vi "Execute.vi"(8 "error in (no error)":errorcluster, 10 "Plugin Handler Launch Plugin in":refnum<class "Plugin Handler Launch Plugin.lvclass">, 11 "Plugin Handler Shifter Data Definition":T1) -> (0 "error out":errorcluster, 1 "Stop?":bool, 2 "Plugin Generic Command out":refnum<class "Plugin Handler Command.lvclass">, 3 "Plugin Handler Shifter Data Out":T1)   [LabVIEW 2011, in "Plugin Handler Launch Plugin.lvclass"]
uses:
  Plugin Handler Launch Plugin.lvclass
  Plugin Handler Command.lvclass
  Plugin Strict Type Definitions/Plugin Handler Shifter Data Definition.ctl
  Parent Plugin Definition/Plugin Template/Generic Plugin.lvclass
  Plugin Strict Type Definitions/Plugin Configuration Information.ctl
  User Interface/UI Command Manager/UI Command Manager.lvclass
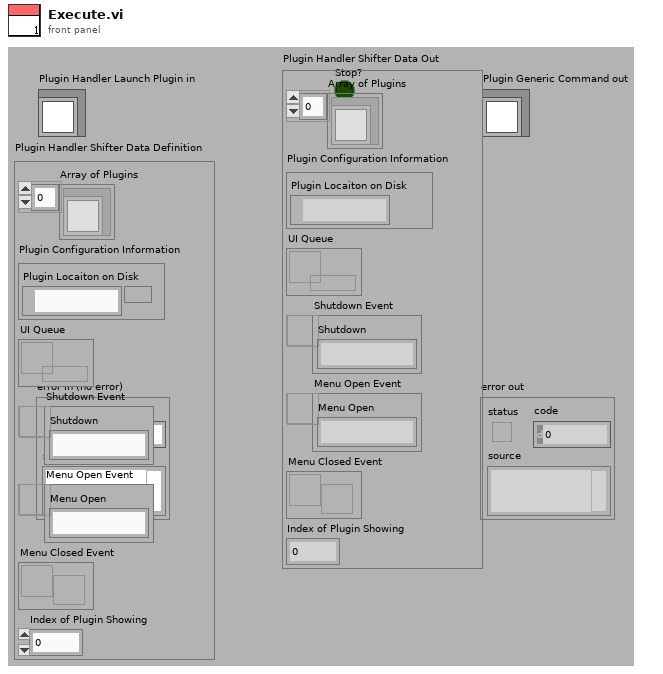
[diagram p1: front panel]
types:
  T1 = typedef "Plugin Handler Shifter Data Definition.ctl" = cluster{"Array of Plugins":refnum<class "Generic Plugin.lvclass">[], "Plugin Configuration Information":T2, "UI Queue":refnum<queue>, "Shutdown Event":refnum<user-event>, "Menu Open Event":refnum<user-event>, "Menu Closed Event":refnum<user-event>, "Index of Plugin Showing":i32}
  T2 = typedef "Plugin Configuration Information.ctl" = cluster{"Plugin Locaiton on Disk":path}
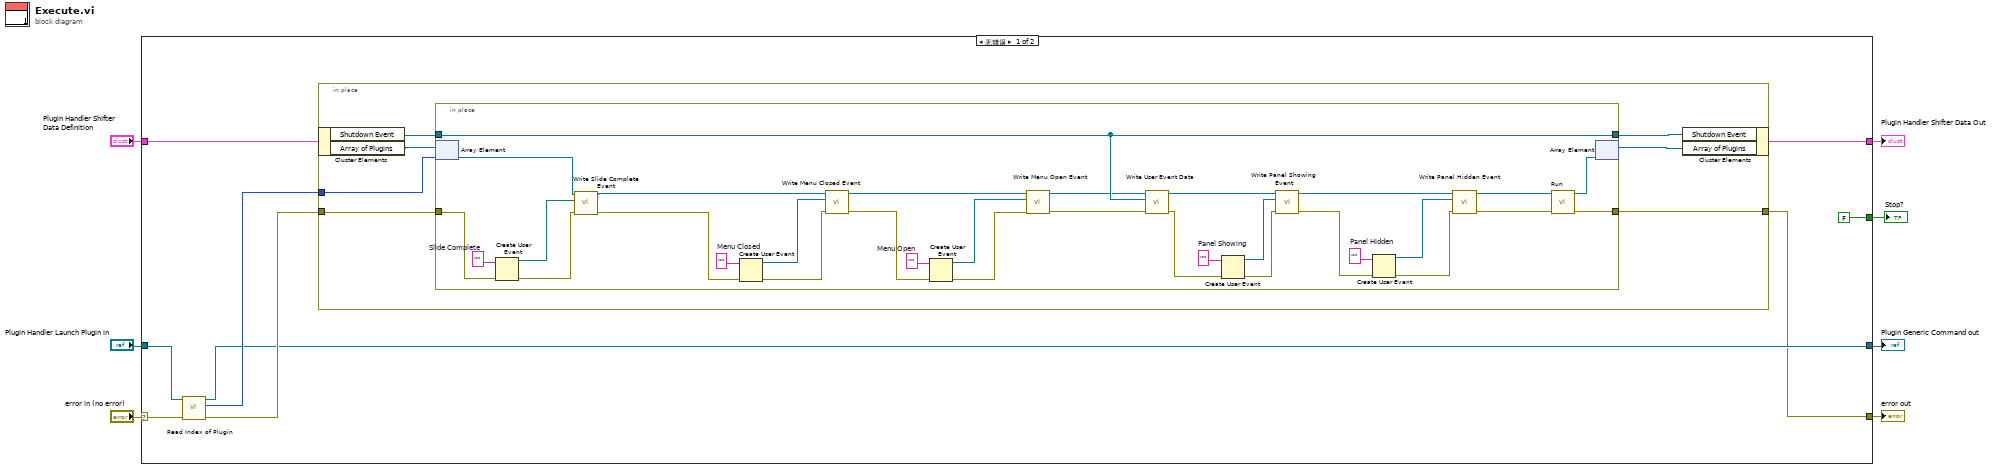
[diagram p0: block diagram]
diagram:
  n1 = case shown="无错误" "error in (no error)" {
    selector: "error in (no error)" -> [w13 w58]
    tunnel: "Plugin Handler Launch Plugin in" -> [w16 w57]
    tunnel: "Plugin Handler Shifter Data Definition" -> [w10 w56]
    tunnel: [w9 w56] -> w5
    tunnel: [w11 w58] -> w3
    tunnel: [w12 w57] -> w2
    tunnel: [FALSE ("Stop?") _] -> w1
    frame No Error {
      n2 = call-dynamic "Read Index of Plugin.vi"("error in (no error)"=w13, "Plugin Handler Launch Plugin in"=w16) -> ("error out"=w14:errorcluster, "Index of Plugin"=w15:i32, "Plugin Handler Launch Plugin out"=w12:refnum<class "Plugin Handler Launch Plugin.lvclass">)  [unwired: 7 in]
      n3 = in-place {
        in-place-border: w15 -> [w20]
        in-place-border: w14 -> [w23]
        in-place-border: [w22] -> w11
        n4 = in-place-cluster #1(w10) -> ("Shutdown Event"=w21:refnum<user-event>, "Array of Plugins"=w18:refnum<class "Generic Plugin.lvclass">[])
        n5 = in-place {
          in-place-border: w23 -> [w32]
          in-place-border: [w50] -> w22
          in-place-border: w21 -> [w55]
          in-place-border: [w55] -> w19
          w33 = ""  # Slide Complete
          w37 = ""  # Menu Open
          w40 = ""  # Menu Closed
          w48 = ""  # Panel Hidden
          w54 = ""  # Panel Showing
          n6 = in-place-array #2(w18, w20) -> (w30:refnum<class "Generic Plugin.lvclass">)
          n7 = Create User Event(user event datatype=w33, error in=w32) -> (user event=w31:refnum<user-event>, error out=w28:errorcluster)
          n8 = call "Write Slide Complete Event.vi"("error in (no error)"=w28, "Slide Complete Event"=w31, "Generic Plugin in"=w30) -> ("error out"=w27:errorcluster, "Generic Plugin out"=w29:refnum<class "Generic Plugin.lvclass">)  [unwired: 7 in]
          n9 = Create User Event(user event datatype=w40, error in=w27) -> (user event=w39:refnum<user-event>, error out=w38:errorcluster)
          n10 = call "Write Menu Closed Event.vi"("error in (no error)"=w38, "Menu Closed Event"=w39, "Generic Plugin in"=w29) -> ("error out"=w35:errorcluster, "Generic Plugin out"=w41:refnum<class "Generic Plugin.lvclass">)  [unwired: 7 in]
          n11 = Create User Event(user event datatype=w37, error in=w35) -> (user event=w36:refnum<user-event>, error out=w34:errorcluster)
          n12 = call "Write Menu Open Event.vi"("error in (no error)"=w34, "Menu Open Event"=w36, "Generic Plugin in"=w41) -> ("error out"=w25:errorcluster, "Generic Plugin out"=w42:refnum<class "Generic Plugin.lvclass">)  [unwired: 7 in]
          n13 = call "Write User Event Data.vi"("error in (no error)"=w25, "User Event Data"=w55, "Generic Plugin in"=w42) -> ("error out"=w24:errorcluster, "Generic Plugin out"=w52:refnum<class "Generic Plugin.lvclass">)  [unwired: 7 in]
          n14 = Create User Event(user event datatype=w54, error in=w24) -> (user event=w53:refnum<user-event>, error out=w26:errorcluster)
          n15 = call "Write Panel Showing Event.vi"("error in (no error)"=w26, "Panel Showing Event"=w53, "Generic Plugin in"=w52) -> ("error out"=w47:errorcluster, "Generic Plugin out"=w49:refnum<class "Generic Plugin.lvclass">)  [unwired: 7 in]
          n16 = Create User Event(user event datatype=w48, error in=w47) -> (user event=w45:refnum<user-event>, error out=w44:errorcluster)
          n17 = call "Write Panel Hidden Event.vi"("error in (no error)"=w44, "Panel Hidden Event"=w45, "Generic Plugin in"=w49) -> ("error out"=w43:errorcluster, "Generic Plugin out"=w46:refnum<class "Generic Plugin.lvclass">)  [unwired: 7 in]
          n18 = call-dynamic "Run.vi"("error in (no error)"=w43, "Generic Plugin in"=w46) -> ("error out"=w50:errorcluster, "Generic Plugin out"=w51:refnum<class "Generic Plugin.lvclass">)  [unwired: 8 in]
          n19 = in-place-array #2(w51) -> (w17:refnum<class "Generic Plugin.lvclass">[])  [unwired: 1 out]
        }
        n20 = in-place-cluster #1("Shutdown Event"=w19, "Array of Plugins"=w17) -> (w9:T1)
      }
    }
    frame Error {
    }
  }
  "error out" <- w3
  "Plugin Generic Command out" <- w2
  "Plugin Handler Shifter Data Out" <- w5
  "Stop?" <- w1
